vi "Transfer Model Resources.vi"(10 "Recipient Model In":refnum<class "IModel.lvclass">, 11 "Running Model":refnum<class "IModel.lvclass">) -> (2 "Recipient Model Out":refnum<class "IModel.lvclass">)   [LabVIEW 2017, in "IModel.lvlib" / "IModel.lvclass"]
uses:
  IModel.lvclass
  C:/Git/mva-framework/Source/Framework/IObserver/IObserver/IObserver.lvclass
  IModel.lvclass/IModel.ctl
  IObserver/IObserver/IObserver.lvclass/IObserver.ctl
  IObserver/IObserver/IObserver.lvclass
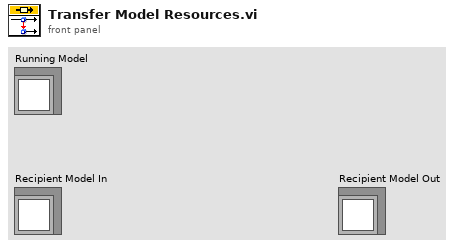
[diagram p1: front panel]
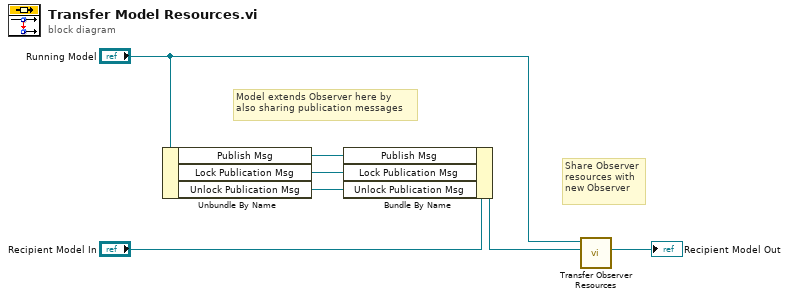
[diagram p0: block diagram]
diagram:
  # "Model extends Observer here by\nalso sharing publication messages"
  # "Share Observer\nresources with\nnew Observer"
  n1 = Unbundle By Name("Running Model") -> ("Publish Msg"=w5:refnum<class "Publish Msg.lvclass">, "Lock Publication Msg"=w6:refnum<class "Lock Publication Msg.lvclass">, "Unlock Publication Msg"=w7:refnum<class "Unlock Publication Msg.lvclass">)
  n2 = Bundle By Name(cluster="Recipient Model In", "Publish Msg"=w5, "Lock Publication Msg"=w6, "Unlock Publication Msg"=w7) -> (w3:refnum<class "IModel.lvclass">)
  n3 = call "Transfer Observer Resources.vi"("Recipient Observer In"=w3, "Running Observer"="Running Model") -> ("Recipient Observer Out"=→"Recipient Model Out":refnum<class "IModel.lvclass">)  [unwired: 9 in]
